vi "Teleop.vi"(10 "Match Info":T1={"Autonomous Elapsed Seconds"=0.0, "TeleOp Elapsed Seconds"=0.0, "Disabled Elapsed Seconds"=0.0, "Visited Autonomous"=FALSE, "Visited TeleOp"=FALSE, "Visited Disabled"=FALSE, "Autonomous Settings"={"Autonomous Style"=enum."Independent", "VI Refnum"=refnum}}, 11 "Call Context":T2) -> ()   [LabVIEW 2016]
doc: "This VI is called for each enabled TeleOp packet received from the DS. It is typically used to read from joysticks and other inputs and update I/O or setpoints for timed control loops. It should complete and return within 20 milliseconds or risk missing DS packets."
uses:
  <vilib>/Rock Robotics/WPI/DriverStation/WPI_DriverStationDerivedRobotMode.ctl
  <vilib>/Rock Robotics/WPI/DriverStation/WPI_DriverStationMatch Info.ctl
  Joystick vals.ctl
  <vilib>/Rock Robotics/WPI/Utilities/WPI_GetSetVariantRefNum.vi
  Framework/Robot Global Data.vi
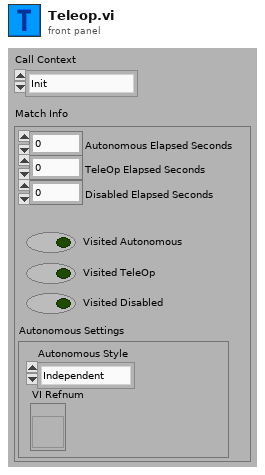
[diagram p1: front panel]
types:
  T1 = typedef "WPI_DriverStationMatch Info.ctl" = cluster{"Autonomous Elapsed Seconds":dbl, "TeleOp Elapsed Seconds":dbl, "Disabled Elapsed Seconds":dbl, "Visited Autonomous":bool, "Visited TeleOp":bool, "Visited Disabled":bool, "Autonomous Settings":cluster{"Autonomous Style":enum16{"Iterative", "Independent"}, "VI Refnum":refnum<vi>}}
  T2 = typedef "WPI_DriverStationDerivedRobotMode.ctl" = enum16{"Init", "Execute", "Stop"}
  T3 = typedef "Joystick vals.ctl" = cluster{"Axes Right":dbl[], " Axes Left":dbl[], " Axes Co-driver":dbl[], "Buttons Right":bool[], "Buttons Left":bool[], "Buttons Co-driver":bool[], "POVs Right":i16[], "POVs Left":i16[], "POVs Co-driver":i16[]}
  T4 = typedef "WPI_JoystickDevRef.ctl" = cluster{"Device":T5}
  T5 = typedef "WPI_JoystickDeviceEnum.ctl" = enum16{"USB 0", "USB 1", "USB 2", "USB 3", "USB 4", "USB 5"}
  T6 = typedef "WPI_MotorControlDeviceRef.ctl" = cluster{"DeviceStatus":errorcluster, "Type":T7, "PWM":cluster{"PWM Channel":T8, "DeadBand":T9}, "CAN":cluster{"Device Number":u8, "SetOutput VI Ref":variant, "GetOutput VI Ref":variant, "Enable VI Ref":variant, "Disable VI Ref":variant, "Data":variant}, "Invert":bool}
  T7 = typedef "WPI_MotorControlType.ctl" = enum16{"PWM", "CAN"}
  T8 = typedef "FPGA_DIOPWMChannel.ctl" = enum8{"PWM 0", "PWM 1", "PWM 2", "PWM 3", "PWM 4", "PWM 5", "PWM 6", "PWM 7", "PWM 8", "PWM 9", "PWM MXP 0", "PWM MXP 1", "PWM MXP 2", "PWM MXP 3", "PWM MXP 4", "PWM MXP 5", "PWM MXP 6", "PWM MXP 7", "PWM MXP 8", "PWM MXP 9", "Invalid"}
  T9 = typedef "WPI_PWMDeadband.ctl" = cluster{"Name":string, "maxPositivePwm":i32, "minPositivePwm":i32, "centerPwm":i32, "maxNegativePwm":i32, "minNegativePwm":i32, "angularRange":u16}
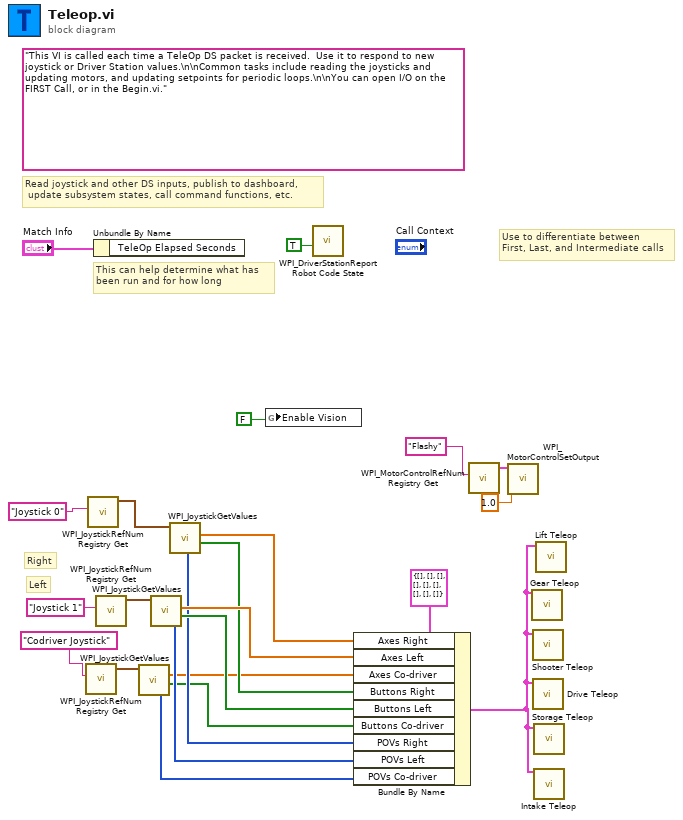
[diagram p0: block diagram]
diagram:
  (unwired) "This VI is called each time a TeleOp DS packet is received.  Use it to respond to new joystick or Driver Station values.\n\nCommon tasks include reading the joysticks and updating motors, and updating setpoints for periodic loops.\n\nYou can open I/O on the FIRST Call, or in the Begin.vi."
  # "Left"
  # "Right"
  # "Read joystick and other DS inputs, publish to dashboard,\n update subsystem states, call command functions, etc."
  # "Use to differentiate between\nFirst, Last, and Intermediate calls"
  # "This can help determine what has\nbeen run and for how long"
  n1 = call <vilib>:"WPI_JoystickRefNum Registry Get.vi"("refnum name"="Codriver Joystick") -> ("JoystickDevRef"=w11:T4)  [unwired: 1 in, 9 out]
  n2 = call <vilib>:"WPI_JoystickRefNum Registry Get.vi"("refnum name"="Joystick 0") -> ("JoystickDevRef"=w20:T4)  [unwired: 1 in, 9 out]
  n3 = Unbundle By Name("Match Info") -> ()  [unwired: 1 out]
  n4 = call <vilib>:"WPI_JoystickRefNum Registry Get.vi"("refnum name"="Joystick 1") -> ("JoystickDevRef"=w19:T4)  [unwired: 1 in, 9 out]
  n5 = call <vilib>:"WPI_JoystickGetValues.vi"("JoystickDevRef"=w11) -> ("Buttons"=w8:bool[], "Axes"=w9:dbl[], "POVs"=w7:i16[])  [unwired: 6 in, 2 out]
  n6 = call <vilib>:"WPI_JoystickGetValues.vi"("JoystickDevRef"=w19) -> ("Buttons"=w14:bool[], "Axes"=w16:dbl[], "POVs"=w12:i16[])  [unwired: 6 in, 2 out]
  n7 = call <vilib>:"WPI_JoystickGetValues.vi"("JoystickDevRef"=w20) -> ("Buttons"=w15:bool[], "Axes"=w17:dbl[], "POVs"=w13:i16[])  [unwired: 6 in, 2 out]
  n8 = global write "Robot Global Data.vi" "Enable Vision"(FALSE) -> ()
  n9 = call <vilib>:"WPI_DriverStationReport Robot Code State.vi"("TeleOp"=TRUE ("Autonomous")) -> ()  [unwired: 10 in, 1 out]
  n10 = Bundle By Name(cluster=T3 {"Axes Right"=[], " Axes Left"=[], " Axes Co-driver"=[], "Buttons Right"=[], "Buttons Left"=[], "Buttons Co-driver"=[], "POVs Right"=[], "POVs Left"=[], "POVs Co-driver"=[]} ("Cluster"), "Axes Right"=w17, "Axes Left"=w16, "Axes Co-driver"=w9, "Buttons Right"=w15, "Buttons Left"=w14, "Buttons Co-driver"=w8, "POVs Right"=w13, "POVs Left"=w12, "POVs Co-driver"=w7) -> (w5:T3)
  n11 = call <vilib>:"WPI_MotorControlRefNum Registry Get.vi"("refnum name"="Flashy") -> ("MotorControlDevRef"=w2:T6)  [unwired: 9 in, 1 out]
  n12 = call <vilib>:"WPI_MotorControlSetOutput.vi"("Output"=1.0, "MotorControlDevRef"=w2) -> ()  [unwired: 7 in, 3 out]
  n13 = call "Gear Teleop.vi"("Cluster"=w5) -> ()  [unwired: 15 in]
  n14 = call "Shooter Teleop.vi"("Cluster"=w5) -> ()  [unwired: 11 in]
  n15 = call "Drive Teleop.vi"("Joystick Vals"=w5) -> ()  [unwired: 11 in]
  n16 = call "Storage Teleop.vi"("Cluster"=w5) -> ()  [unwired: 11 in]
  n17 = call "Intake Teleop.vi"("Cluster"=w5) -> ()  [unwired: 15 in]
  n18 = call "Lift Teleop.vi"("Cluster"=w5) -> ()  [unwired: 11 in]
